vi "Generate AO Waveforms.vi"(6 "reset phase":bool, 8 "error in (no error)":errorcluster, 11 "Generator in":refnum<class "Generator.lvclass">) -> (0 "error out":errorcluster, 2 "AO Array":waveform(dbl)[](array[waveform]), 3 "Generator out":refnum<class "Generator.lvclass">, 4 "phase reset":bool)   [LabVIEW 2019, in "Generator.lvclass"]
uses:
  Generator.lvclass
  typedefs/AO.Channel--Cluster--Array.ctl
  typedefs/AO.Channel--Cluster.ctl
  typedefs/AO.Channel.Function--Enum.ctl
  Generator.lvclass/Generator.ctl
  <vilib>/Waveform/WDTOps.llb/WDT Append Waveforms DBL.vi
  <vilib>/measure/NI_MABase.lvlib
panel:
  in  "Tab Control":enum32{"Page 1", "Graphs"}(tab)
  out "AO Channels":T1 {"Duty Cycle" format="%.3g"; "Phase" format="%.3g"; "Frequency" min=0.0001 max=10000.0 format="%.3g"; "Offset" format="%5.2p"; "Amplitude" min=0.0 max=10.0 format="%5.2p"}
  out "Waveform Graph":waveform(dbl)[](graph)
  out "Phase Chart":dbl[][](graph)
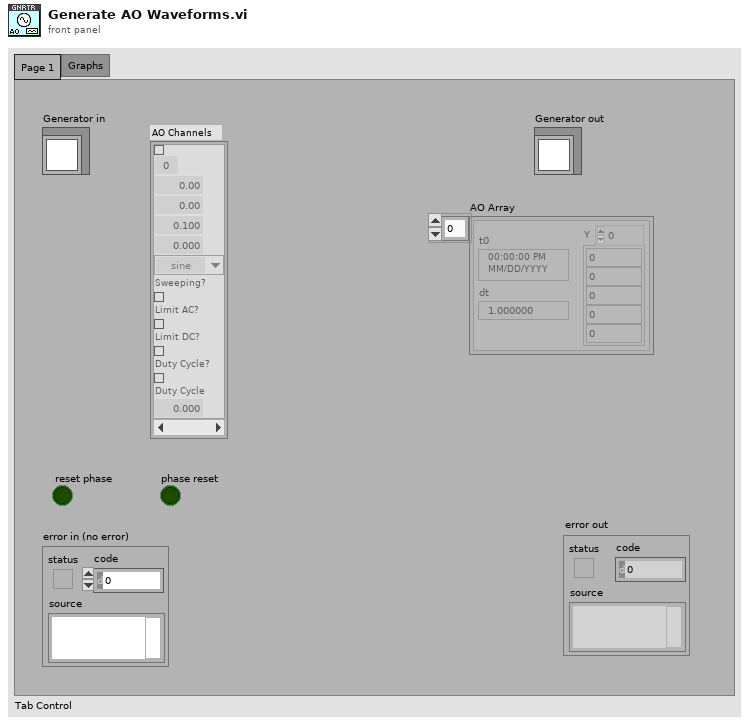
[diagram p1: front panel]
types:
  T1 = typedef "Generator.lvclass/AO.Channel--Cluster--Array.ctl" = T2[]
  T2 = typedef "Generator.lvclass/AO.Channel--Cluster.ctl" = cluster{"Enable?":bool, "Channel":i32, "Amplitude":dbl, "Offset":dbl, "Frequency":dbl, "Phase":dbl, "Function":T3, "Sweeping?":bool, "Limit AC?":bool, "Limit DC?":bool, "Duty Cycle?":bool, "Duty Cycle":dbl}
  T3 = typedef "Generator.lvclass/AO.Channel.Function--Enum.ctl" = enum16{"sine", "square", "triangle", "saw"}
  T4 = enum16{"Sine Wave", "Triangle Wave", "Square Wave", "Sawtooth Wave"}
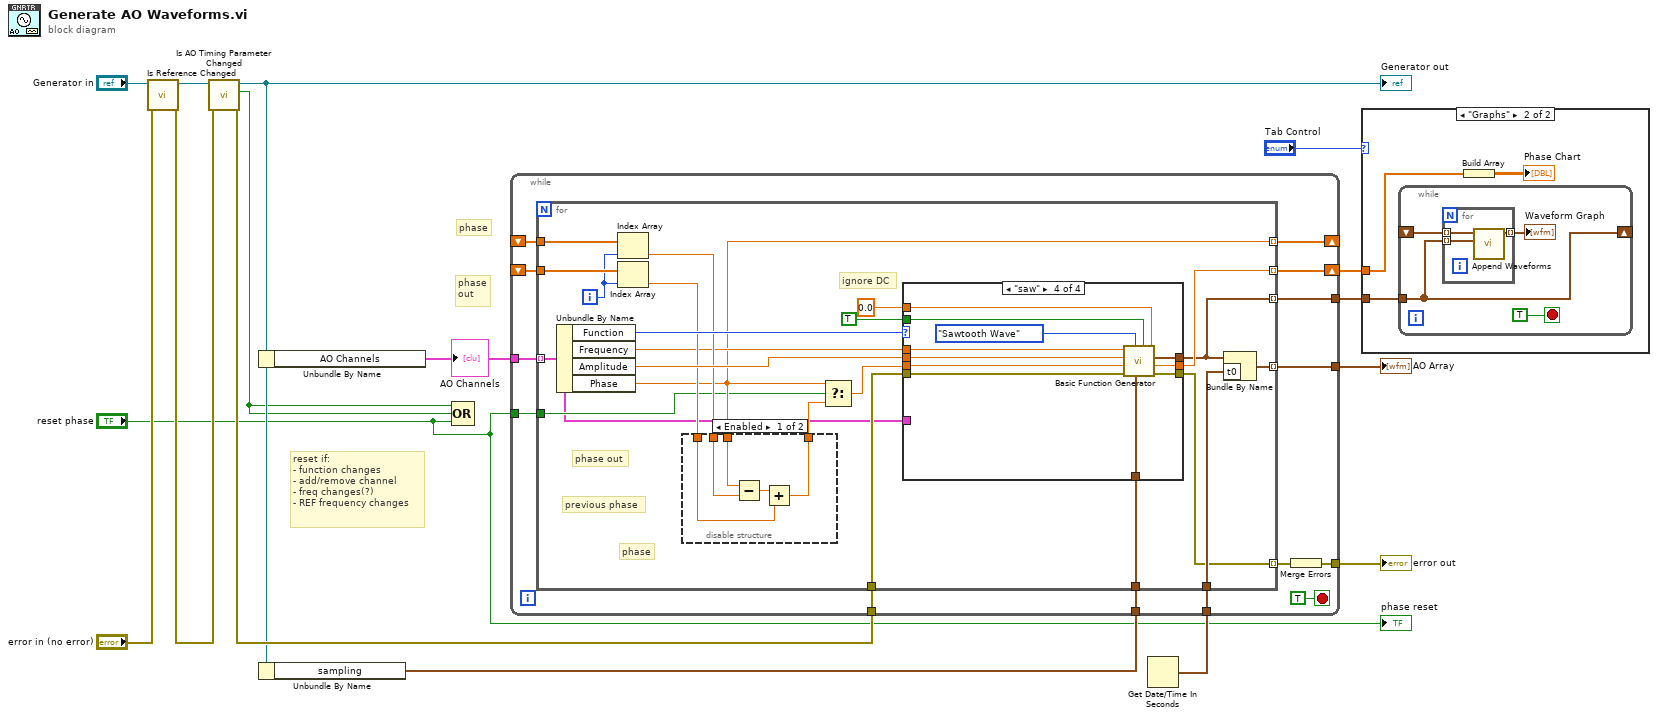
[diagram p0: block diagram]
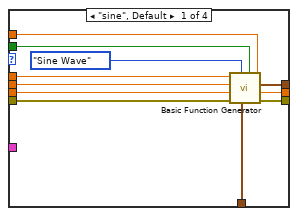
[diagram p3: hidden frame]
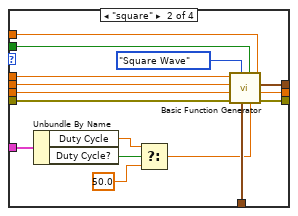
[diagram p4: hidden frame]
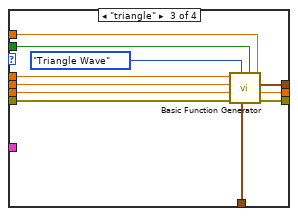
[diagram p5: hidden frame]
diagram:
  # "phase"
  # "phase\nout"
  # "reset if:\n- function changes\n- add/remove channel\n- freq changes(?)\n- REF frequency changes"
  n1 = call "Is Reference Changed.vi"("error in (no error)"="error in (no error)", "Generator in"="Generator in") -> ("error out"=w6:errorcluster, "Generator out"=w7:refnum<class "Generator.lvclass">)  [unwired: 7 in, 1 out]
  n2 = call "Is AO Timing Parameter Changed.vi"("error in (no error)"=w6, "Generator in"=w7) -> ("error out"=w5:errorcluster, "AO frequency or phase or function changed?"=w2:bool, "Generator out"=w3:refnum<class "Generator.lvclass">)  [unwired: 7 in]
  "Generator out" <- w3
  n3 = Unbundle By Name(w3) -> ("AO Channels"=w10:T1)
  "AO Channels" <- w10
  n4 = Unbundle By Name(w3) -> ("sampling"=w8:cluster{"Fs":dbl, "#s":dbl})
  n5 = Compound Arithmetic op=OR(w2, w2, "reset phase") -> ()  [unwired: 1 out]
  n6 = Get Date/Time In Seconds() -> (seconds since 1Jan1904=w16:timestamp)
  n7 = while {
    tunnel: w8 -> [w30]
    tunnel: [w29] -> w14
    shift-right: [w27] -> w13
    shift-left: _ -> [w19]
    tunnel: w16 -> [w26]
    tunnel: w5 -> [w25]
    tunnel: [w23] -> w15
    tunnel: w10 -> [w22]
    shift-right: [w21] -> _
    shift-left: _ -> [w18]
    tunnel: [w20] -> w12
    tunnel: "reset phase" -> [w17]
    stop <- TRUE stop-if-true
    n8 = for {
      tunnel: [w50] -> w29 mode=indexing
      tunnel: w30 -> [w48]
      tunnel: [w37] -> w27 mode=indexing
      tunnel: w26 -> [w52]
      tunnel: w25 -> [w46]
      tunnel: [w49] -> w24 mode=indexing
      tunnel: w22 -> [w31] mode=indexing
      tunnel: w19 -> [w43]
      tunnel: [w34] -> w21 mode=indexing
      tunnel: w18 -> [w39]
      tunnel: [w36] -> w20 mode=indexing
      tunnel: w17 -> [w33]
      i -> [w42]
      # "previous phase"
      # "phase"
      # "phase out"
      # "ignore DC"
      n9 = Unbundle By Name(w31) -> ("Function"=w44:T3, "Frequency"=w35:dbl, "Amplitude"=w45:dbl, "Phase"=w34:dbl)
      n10 = Index Array(array=w39, index=w42) -> (element=w40:dbl)
      n11 = Index Array(array=w43, index=w42) -> (element=w41:dbl)
      n12 = disable-structure shown="Enabled" {
        disable-tunnel: w34 -> [w57 _]
        disable-tunnel: w40 -> [w56 _]
        disable-tunnel: w41 -> [w53 w58]
        disable-tunnel: [w55 w58] -> w32
        frame Enabled {
          n13 = Subtract(x=w57, y=w56) -> (x-y=w54:dbl)
          n14 = Add(x=w54, y=w53) -> (x+y=w55:dbl)
        }
        frame Disabled {
        }
      }
      n15 = Select(t=w34, s=w33, f=w32) -> (s? t:f=w38:dbl)
      n16 = case shown="\"saw\"" w44 {
        tunnel: w35 -> [w69 w85 w96 w107]
        tunnel: 0.0 ("AO DC") -> [w68 w84 w95 w106]
        tunnel: [w67 w83 w94 w105] -> w36
        tunnel: TRUE ("reset signal") -> [w59 w75 w86 w97]
        tunnel: w46 -> [w66 w82 w93 w104]
        tunnel: [w65 w81 w92 w103] -> w49
        tunnel: [w64 w80 w91 w102] -> w37
        tunnel: w45 -> [w63 w79 w90 w101]
        tunnel: w38 -> [w62 w78 w89 w100]
        tunnel: w48 -> [w61 w77 w88 w99]
        tunnel: w31 -> [_ w72 _ _]
        frame "sine", Default {
          n17 = call <vilib>:"Basic Function Generator.vi"("offset"=w68, "reset signal"=w59, "sampling info"=w61, "signal type"=T4."Sine Wave", "error in (no error)"=w66, "phase"=w62, "amplitude"=w63, "frequency"=w69) -> ("error out"=w65:errorcluster, "phase out"=w64:dbl, "signal out"=w67:waveform(dbl))  [unwired: 1 in]
        }
        frame "square" {
          n18 = Unbundle By Name(w72) -> ("Duty Cycle"=w70:dbl, "Duty Cycle?"=w74:bool)
          n19 = Select(t=w70, s=w74, f=50.0) -> (s? t:f=w71:dbl)
          n20 = call <vilib>:"Basic Function Generator.vi"("offset"=w84, "square wave duty cycle (%)"=w71, "reset signal"=w75, "sampling info"=w77, "signal type"=T4."Square Wave", "error in (no error)"=w82, "phase"=w78, "amplitude"=w79, "frequency"=w85) -> ("error out"=w81:errorcluster, "phase out"=w80:dbl, "signal out"=w83:waveform(dbl))
        }
        frame "triangle" {
          n21 = call <vilib>:"Basic Function Generator.vi"("offset"=w95, "reset signal"=w86, "sampling info"=w88, "signal type"=T4."Triangle Wave", "error in (no error)"=w93, "phase"=w89, "amplitude"=w90, "frequency"=w96) -> ("error out"=w92:errorcluster, "phase out"=w91:dbl, "signal out"=w94:waveform(dbl))  [unwired: 1 in]
        }
        frame "saw" {
          n22 = call <vilib>:"Basic Function Generator.vi"("offset"=w106, "reset signal"=w97, "sampling info"=w99, "signal type"=T4."Sawtooth Wave", "error in (no error)"=w104, "phase"=w100, "amplitude"=w101, "frequency"=w107) -> ("error out"=w103:errorcluster, "phase out"=w102:dbl, "signal out"=w105:waveform(dbl))  [unwired: 1 in]
        }
      }
      n23 = Bundle By Name(cluster=w36, "t0"=w52) -> (w50:waveform(dbl))
    }
    n24 = Merge Errors(w24) -> (w23:errorcluster)
  }
  "AO Array" <- w14
  "error out" <- w15
  n25 = case shown="\"Graphs\"" "Tab Control" {
    tunnel: w12 -> [_ w108]
    tunnel: w13 -> [_ w109]
    frame Default {
    }
    frame "Graphs" {
      n26 = while {
        shift-right: [w111] -> _
        shift-left: _ -> [w112]
        tunnel: w108 -> [w111]
        stop <- TRUE stop-if-true
        n27 = for {
          tunnel: [w117] -> w113 mode=indexing
          tunnel: w112 -> [w116] mode=indexing
          tunnel: w111 -> [w115] mode=indexing
          n28 = call-poly <vilib>:"Append Waveforms.vi"("waveform B"=w115, "waveform A"=w116) -> ("waveform out"=w117:waveform(dbl))  [unwired: 8 in, 1 out]
        }
        "Waveform Graph" <- w113
      }
      n29 = Build Array(w109) -> (→"Phase Chart":dbl[][])
    }
  }
  "phase reset" <- "reset phase"
